vi "VI under test.vi"(10 "x":dbl, 11 "y":dbl) -> (3 "x+y":dbl)   [LabVIEW 2020, in "Test Vector Demo.lvclass"]
uses:
  Test Vector Demo.lvclass
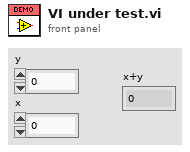
[diagram p1: front panel]
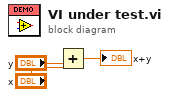
[diagram p0: block diagram]
diagram:
  n1 = Add(x="x", y="y") -> (x+y=→"x+y":dbl)
